vi "Animal Data Processor.vi"() -> (0 "Data Export":T1 {"Data Channels" format="%.2f"})   [LabVIEW 2016]
uses:
  Animal Data Processor state.ctl
  <vilib>/regexp/Match Regular Expression.xnode
panel:
  in  "Case Constant\n(See Context Help)":bool
  in  "Number of Impulse Files":i32
  in  "Field Strengths":i32[](array[numeric])=[1, 2, 7, 8, 13, 14, 20]
  in  "Impulse Data File (auto increment)":bool
  in  "Field Gains from File":bool
  in  "All Data":T1 {"Data Channels" format="%.2f"}
  in  "Tab Control":enum32{"Channel Information", "Default Values"}(tab)
  in  "Defaults":bool
  in  "Coil Combinations":T2(array[cluster])=[{"Direction Coil"=0, "Torsion Coil"=0, "Dir"=FALSE, "tor"=FALSE}, {"Direction Coil"=0, "Torsion Coil"=2, "Dir"=TRUE, "tor"=TRUE}, {"Direction Coil"=2, "Torsion Coil"=3, "Dir"=TRUE, "tor"=TRUE}]
  in  "Coil Information":T3(array[cluster])=[{"X Field"={"Channel No."=2, "Peak Field "=911, "Offset"=0.0, "Gain"=0.0625}, "Y Field"={"Channel No."=0, "Peak Field "=-904, "Offset"=0.0, "Gain"=0.0625}, "Z Field"={"Channel No."=1, "Peak Field "=961, "Offset"=0.0, "Gain"=0.0625}}, {"X Field"={"Channel No."=5, "Peak Field "=770, "Offset"=0.0, "Gain"=0.0625}, "Y Field"={"Channel No."=3, "Peak Field "=-723, "Offset"=0.0, "Gain"=0.0625}, "Z Field"={"Channel No."=4, "Peak Field "=771, "Offset"=0.0, "Gain"=0.0625}}, {"X Field"={"Channel No."=8, "Peak Field "=603, "Offset"=0.0, "Gain"=0.0625}, "Y Field"={"Channel No."=6, "Peak Field "=-647, "Offset"=0.0, "Gain"=0.0625}, "Z Field"={"Channel No."=7, "Peak Field "=627, "Offset"=0.0, "Gain"=0.0625}}, {"X Field"={"Channel No."=11, "Peak Field "=1030, "Offset"=0.0, "Gain"=0.0625}, "Y Field"={"Channel No."=9, "Peak Field "=-1108, "Offset"=0.0, "Gain"=0.0625}, "Z Field"={"Channel No."=10, "Peak Field "=1074, "Offset"=0.0, "Gain"=0.0625}}] {"Z Field"."Gain" format="%.4f"; "Z Field"."Offset" format="%.2f"; "Y Field"."Gain" format="%.4f"; "Y Field"."Offset" format="%.2f"; "X Field"."Gain" format="%.4f"; "X Field"."Offset" format="%.2f"}
  in  "Additional Channels":T4(array[cluster])=[{"Channel No."=12, "Scaling Factor"=0.00030518, "Channel Name"=0, "Offset Factor"=0, "Acutrol Cal"=20}, {"Channel No."=13, "Scaling Factor"=0.00030518, "Channel Name"=1, "Offset Factor"=0, "Acutrol Cal"=20}, {"Channel No."=14, "Scaling Factor"=0.00030518, "Channel Name"=2, "Offset Factor"=0, "Acutrol Cal"=20}, {"Channel No."=15, "Scaling Factor"=0.00030518, "Channel Name"=3, "Offset Factor"=0, "Acutrol Cal"=20}] {"Acutrol Cal" min=0 max=40 step=20; "Channel Name" items=["Chair Position", "Chair Velocity", "Sled Position", "Sled Velocity"]; "Scaling Factor" format="%.4e"}
  in  "Available Channel Names":string[](array[string])=["Chair Position", "Chair Velocity", "Sled Position", "Sled Velocity"]
  in  "Data File":T5 {"Data -> Additional" format="%.2f"; "Data -> 3D Coil" format="%.2f"}
  in  "For DY DZ  (H LE RE) plot\n                 Channel No.":i32[](array[numeric])=[1, 2, 7, 8, 13, 14, 18]
  in  "Export Channel List":u16[](array[ring])=[3, 4, 5, 14, 15, 16, 17, 18, 29, 30, 31, 32, 33, 6, 7, 8, 19, 20, 21, 22, 23, 34, 35, 36, 37, 38, 39, 40, 41, 42, 43] items=["Hx Position-in-Space", "Hy Position-in-Space", "Hz Position-in-Space", "Lx Position-in-Space", "Ly Position-in-Space", "Lz Position-in-Space", "Rx Position-in-Space", "Ry Position-in-Space", "Rz Position-in-Space", "Hx Velocity-in-Space", "Hy Velocity-in-Space", "Hz Velocity-in-Space", "Hl Velocity-in-Space", "Hr Velocity-in-Space", "Lx Velocity-in-Space", "Ly Velocity-in-Space", "Lz Velocity-in-Space", "Ll Velocity-in-Space", "Lr Velocity-in-Space", "Rx Velocity-in-Space", "Ry Velocity-in-Space", "Rz Velocity-in-Space", "Rl Velocity-in-Space", "Rr Velocity-in-Space", "Hx Acceleration-in-Space", "Hy Acceleration-in-Space", "Hz Acceleration-in-Space", "Hl Acceleration-in-Space", "Hr Acceleration-in-Space", "Lx Acceleration-in-Space", "Ly Acceleration-in-Space", "Lz Acceleration-in-Space", "Ll Acceleration-in-Space", "Lr Acceleration-in-Space", "Rx Acceleration-in-Space", "Ry Acceleration-in-Space", "Rz Acceleration-in-Space", "Rl Acceleration-in-Space", "Rr Acceleration-in-Space", "Chair Position", "Chair Velocity", "Sled Position", "Sled Velocity", " "]
  out "Processing":bool
  in  "Start Processing":bool
  in  "Selected Data File":string
  in  "Data File":bool
  in  "Quit":bool
  in  "Stop":bool
  # "Animal Data Processor"
  # "AAM 10 april 2002 ver.10"
  # "Copyright Americo A. Migliaccio (c) 2002 All Rights Reserved by Author"
  # "NOTE: EMPTY LIST ALWAYS AT END"
  # "Head 0; Left Eye 1; Right Eye 2"
  # "Name                        Channel            Offset            Gain               Acutrol Cal"
  # "Channel            Field               Offset             Gain"
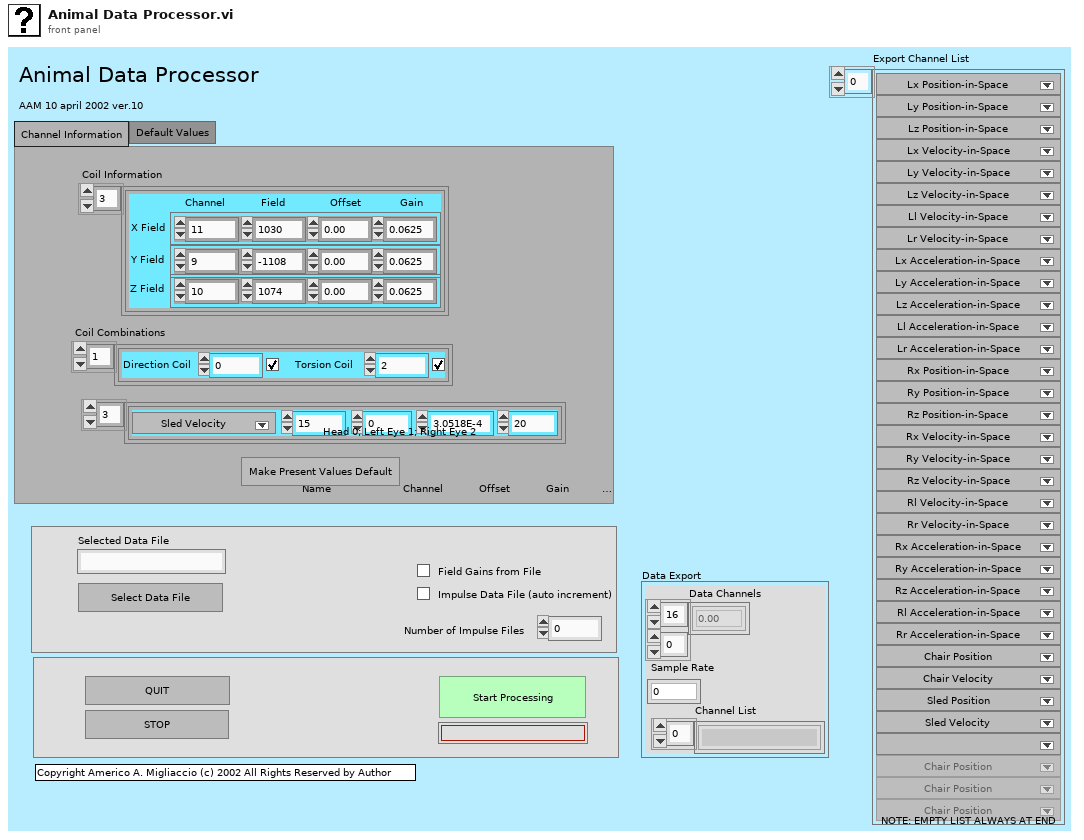
[diagram p1: front panel]
types:
  T1 = cluster{"Data Channels":dbl[][], "Sample Rate":i32, "Channel List":string[]}
  T2 = cluster{"Direction Coil":i32, "Torsion Coil":i32, "Dir":bool, "tor":bool}[]
  T3 = cluster{"X Field":cluster{"Channel No.":i32, "Peak Field ":i32, "Offset":dbl, "Gain":dbl}, "Y Field":cluster{"Channel No.":i32, "Peak Field ":i32, "Offset":dbl, "Gain":dbl}, "Z Field":cluster{"Channel No.":i32, "Peak Field ":i32, "Offset":dbl, "Gain":dbl}}[]
  T4 = cluster{"Channel No.":i32, "Scaling Factor":dbl, "Channel Name":u16, "Offset Factor":i32, "Acutrol Cal":i32}[]
  T5 = cluster{"No. Channels":i32, "Sample Rate":i32, "Data -> 3D Coil":dbl[][], "Data -> Additional":dbl[][]}
  T6 = typedef "Animal Data Processor state.ctl" = enum16{"Calculate 6 Field/Int Rot Matrix", "Panel Monitoring", "Initialize", "Read 6 Field/Int Calibration File", "Read 6 Field/Int Data File", "Sort 6 Field/Int Channels", "Export Channels", "Stop", "Quit"}
  T7 = enum16{"open", "open or create", "create or replace", "create", "open (read only)"}
  T8 = enum16{"Position in Space", "Position in Head", "Position in Eye", "Velocity in Space", "Velocity in Head", "Velocity in Eye", "Acceleration in Space", "Acceleration in Head"}
  T9 = cluster{"Coil Information":cluster{"X Field":cluster{"Channel No.":i32, "Peak Field ":i32, "Offset":dbl, "Gain":dbl}, "Y Field":cluster{"Channel No.":i32, "Peak Field ":i32, "Offset":dbl, "Gain":dbl}, "Z Field":cluster{"Channel No.":i32, "Peak Field ":i32, "Offset":dbl, "Gain":dbl}}[], "Coil Combinations":cluster{"Direction Coil":i32, "Torsion Coil":i32, "Dir":bool, "tor":bool}[], "Additional Channels":cluster{"Channel No.":i32, "Scaling Factor":dbl, "Channel Name":u16, "Offset Factor":i32, "Acutrol Cal":i32}[], "Selected Data File":string, "Data File":cluster{"No. Channels":i32, "Sample Rate":i32, "Data -> 3D Coil":dbl[][], "Data -> Additional":dbl[][]}, "For DY DZ  (H LE RE) plot\n                 Channel No.":i32[], "All Data":cluster{"Data Channels":dbl[][], "Sample Rate":i32, "Channel List":string[]}, "Field Strengths":i32[]}
  T10 = cluster{"Stop ":bool, "Quit":bool, "Data File":bool, "Start Processing":bool, "Defaults":bool}
  T11 = cluster{"Coil Information":cluster{"X Field":cluster{"Channel No.":i32, "Peak Field ":i32, "Offset":dbl, "Gain":dbl}, "Y Field":cluster{"Channel No.":i32, "Peak Field ":i32, "Offset":dbl, "Gain":dbl}, "Z Field":cluster{"Channel No.":i32, "Peak Field ":i32, "Offset":dbl, "Gain":dbl}}[], "Coil Combinations":cluster{"Direction Coil":i32, "Torsion Coil":i32, "Dir":bool, "tor":bool}[], "Additional Channels":cluster{"Channel No.":i32, "Scaling Factor":dbl, "Channel Name":u16, "Offset Factor":i32, "Acutrol Cal":i32}[]}
  T12 = cluster{"X Field":cluster{"Channel No.":i32, "Peak Field ":i32, "Offset":dbl, "Gain":dbl}, "Y Field":cluster{"Channel No.":i32, "Peak Field ":i32, "Offset":dbl, "Gain":dbl}, "Z Field":cluster{"Channel No.":i32, "Peak Field ":i32, "Offset":dbl, "Gain":dbl}}
  T13 = enum16{"Rotation Matrix", "Rotation Vectors", "Quaternions", "Fick Angles", "Helmholtz Angles"}
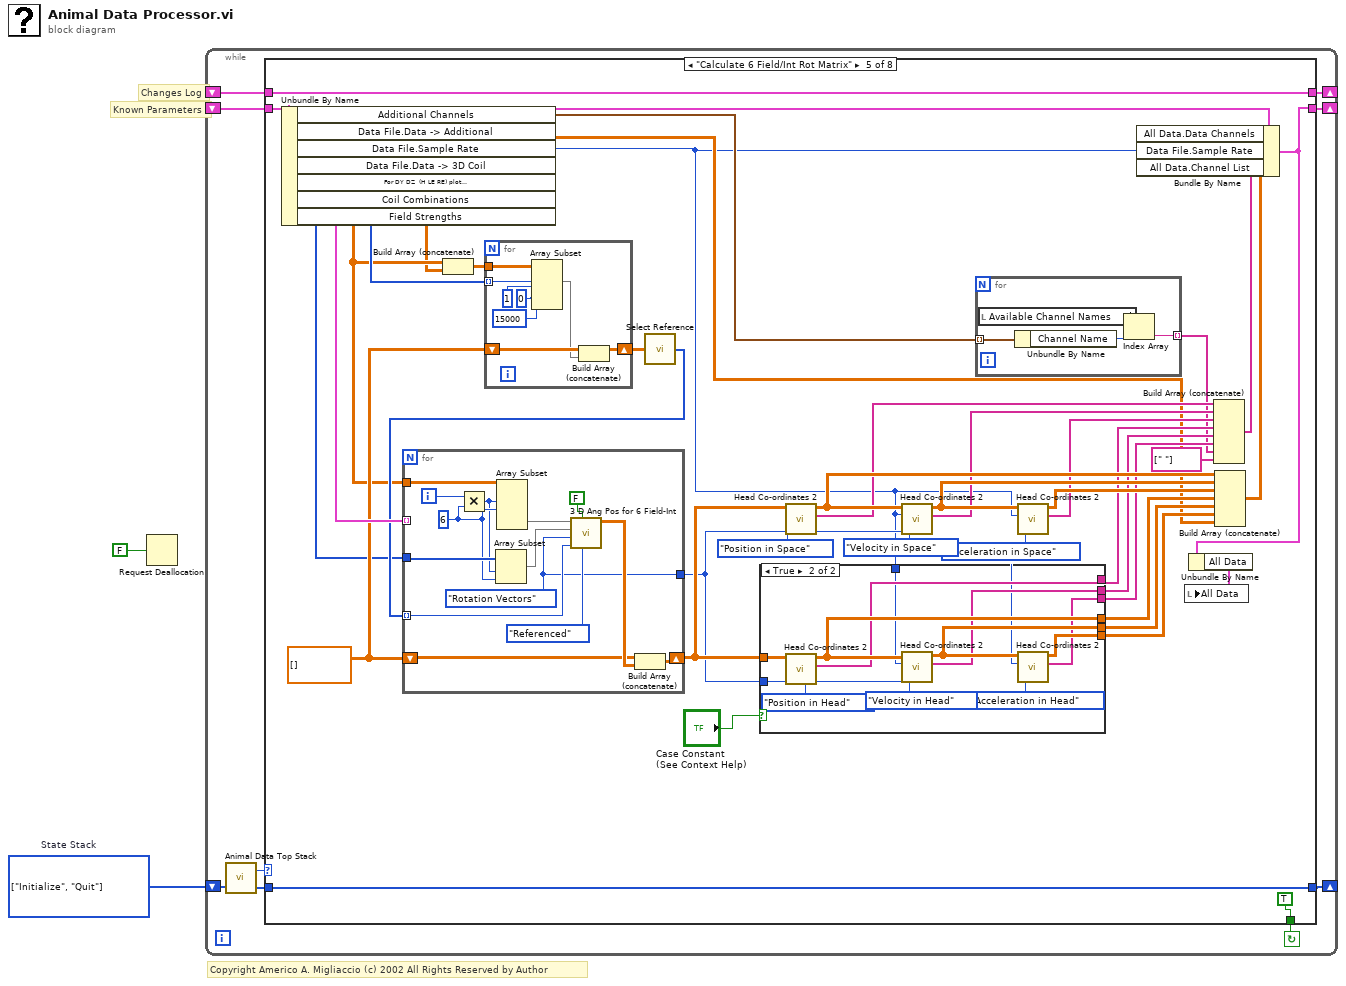
[diagram p0: block diagram]
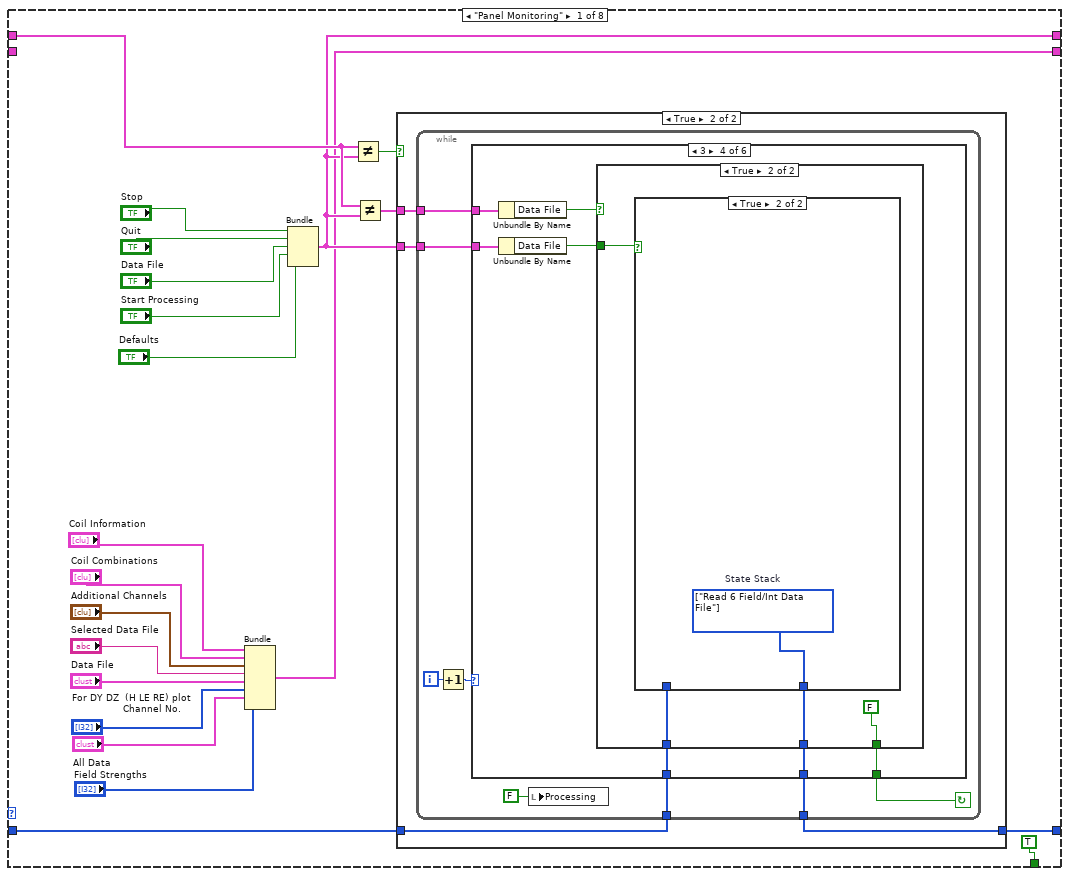
[diagram p2: hidden frame]
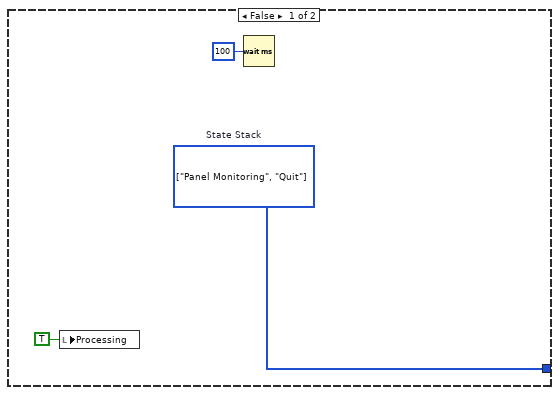
[diagram p3: hidden frame]
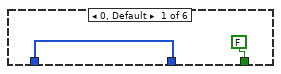
[diagram p4: hidden frame]
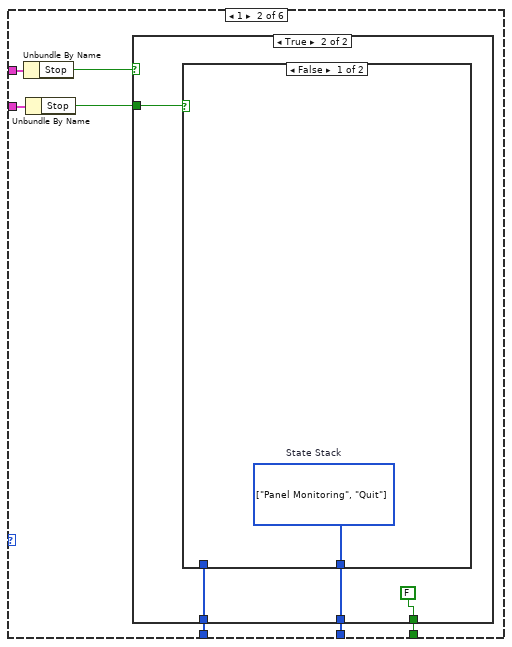
[diagram p5: hidden frame]
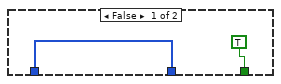
[diagram p6: hidden frame]
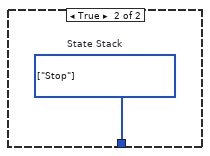
[diagram p7: hidden frame]
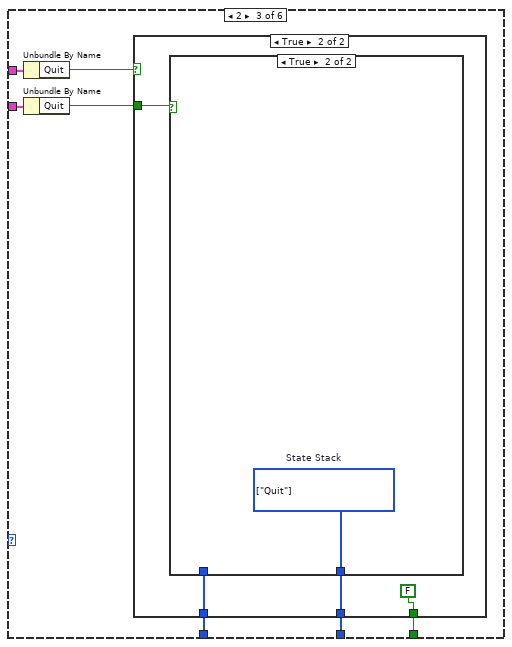
[diagram p8: hidden frame]
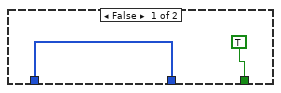
[diagram p9: hidden frame]
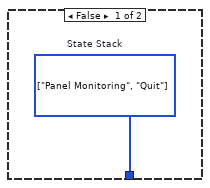
[diagram p10: hidden frame]
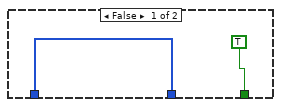
[diagram p11: hidden frame]
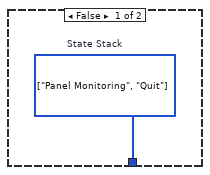
[diagram p12: hidden frame]
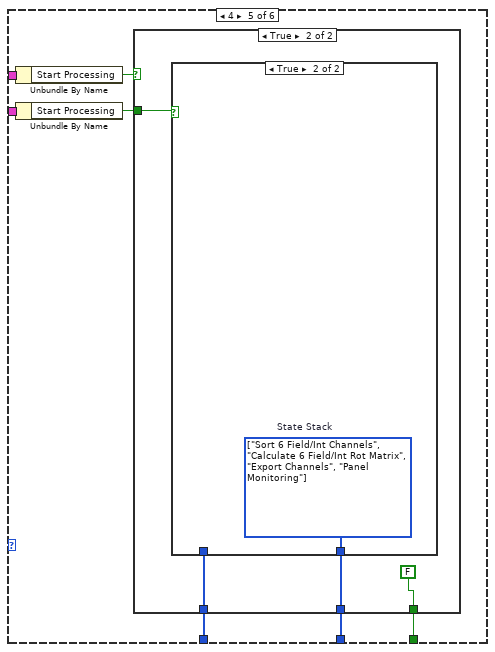
[diagram p13: hidden frame]
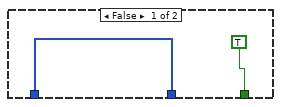
[diagram p14: hidden frame]
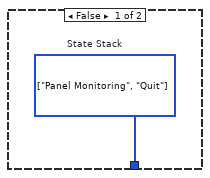
[diagram p15: hidden frame]
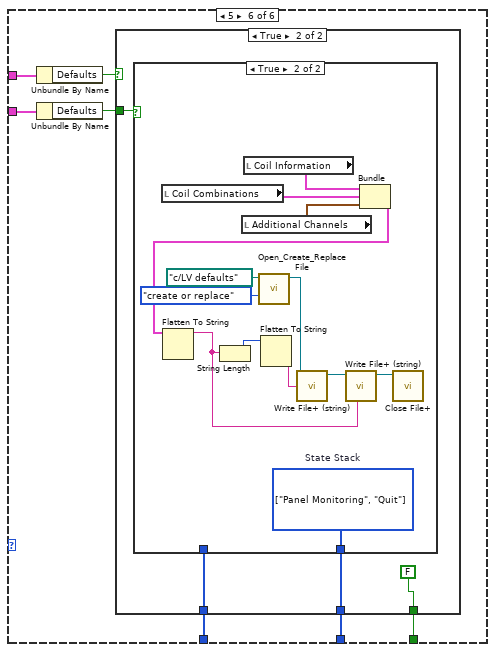
[diagram p16: hidden frame]
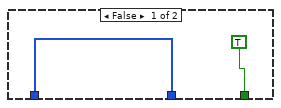
[diagram p17: hidden frame]
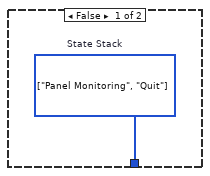
[diagram p18: hidden frame]
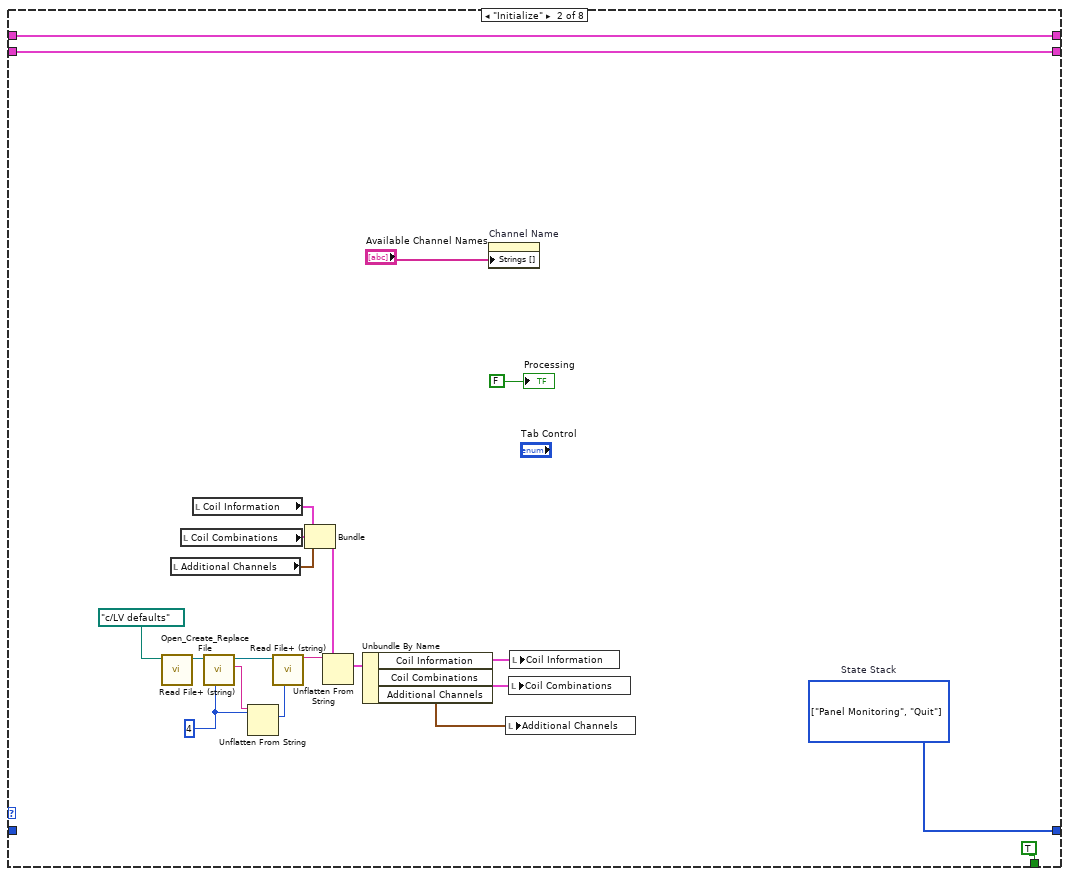
[diagram p19: hidden frame]
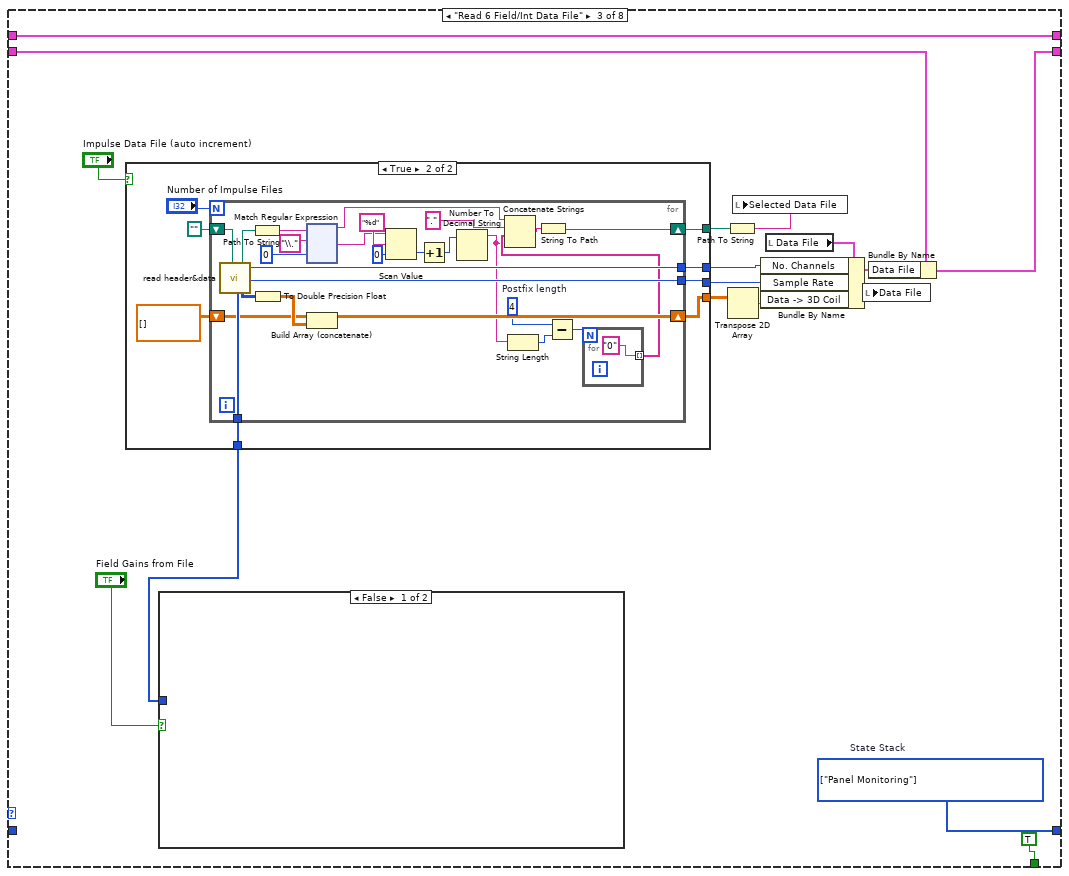
[diagram p20: hidden frame]
diagram:
  w2 = T6[] [enum."Initialize", enum."Quit"] items=["Calculate 6 Field/Int Rot Matrix", "Panel Monitoring", "Initialize", "Read 6 Field/Int Calibration File", "Read 6 Field/Int Data File", "Sort 6 Field/Int Channels", "Export Channels", "Stop", "Quit"]  # State Stack
  # "Copyright Americo A. Migliaccio (c) 2002 All Rights Reserved by Author"
  # "Known Parameters"
  # "Changes Log"
  n1 = Request Deallocation(FALSE ("flag")) -> ()
  n2 = while {
    shift-left: _ -> [w4]
    shift-right: [w3] -> _
    shift-left: _ -> [w6]
    shift-right: [w7] -> _
    shift-left: w2 -> [w11]
    shift-right: [w9] -> _
    stop <- w5 continue-if-true
    n3 = call "Animal Data Top Stack.vi"("State Stack (in)"=w11) -> ("State Stack (out)"=w10:T6[], "State"=w8:T6)  [unwired: 1 in]
    n4 = case shown="\"Calculate 6 Field/Int Rot Matrix\"" w8 {
      tunnel: w10 -> [w27 _ _ w353 w489 w541 w550 w554]
      tunnel: [w26 w153 w169 w353 w489 w541 w550 w554] -> w9
      tunnel: [w24 w156 w172 w355 w487 w539 w548 w552] -> w7
      tunnel: w6 -> [w29 w156 w172 w355 w487 w539 w548 w552]
      tunnel: [TRUE TRUE TRUE TRUE TRUE FALSE FALSE FALSE] -> w5
      tunnel: [w12 w145 w171 w352 w471 w535 w547 w551] -> w3
      tunnel: w4 -> [_ w145 w170 w354 w481 w535 w547 w551]
      frame "Panel Monitoring" {
        n5 = Bundle("Coil Information"="Coil Information", "Coil Combinations"="Coil Combinations", "Additional Channels"="Additional Channels", "Selected Data File"="Selected Data File", "Data File"="Data File", "For DY DZ  (H LE RE) plot\n                 Channel No."="For DY DZ  (H LE RE) plot\n                 Channel No.", "All Data"="All Data", "Field Strengths"="Field Strengths") -> (w12:T9)  [unwired: 1 in]
        n6 = Bundle("Stop"="Stop", "Quit"="Quit", "Data File"="Data File", "Start Processing"="Start Processing", "Defaults"="Defaults") -> (w24:T10)  [unwired: 1 in]
        n7 = Not Equal?(x=w29, y=w24) -> (x != y?=w30:bool)
        n8 = Not Equal?(x=w29, y=w24) -> (x != y?=w28:T10)
        n9 = case shown="True" w30 {
          tunnel: w28 -> [_ w39]
          tunnel: w27 -> [_ w37]
          tunnel: [w33 w38] -> w26
          tunnel: w24 -> [_ w36]
          frame False {
            w33 = T6[] [enum."Panel Monitoring", enum."Quit"] items=["Calculate 6 Field/Int Rot Matrix", "Panel Monitoring", "Initialize", "Read 6 Field/Int Calibration File", "Read 6 Field/Int Data File", "Sort 6 Field/Int Channels", "Export Channels", "Stop", "Quit"]  # State Stack
            n10 = local write "Processing"(TRUE ("Processing")) -> ()
            n11 = Wait (ms)(milliseconds to wait=u32 100) -> ()  [unwired: 1 out]
          }
          frame True {
            n12 = while {
              tunnel: w36 -> [w41]
              tunnel: w37 -> [w44]
              tunnel: [w45] -> w38
              tunnel: w39 -> [w47]
              i -> [w46]
              stop <- w43 continue-if-true
              n13 = Increment(x=w46) -> (x+1=w42:i32)
              n14 = case shown="3" w42 {
                tunnel: w47 -> [_ w56 w71 w86 w101 w116]
                tunnel: [w49 w54 w69 w84 w99 w114] -> w45
                tunnel: w44 -> [w49 w53 w68 w83 w98 w113]
                tunnel: [FALSE w52 w67 w82 w97 w112] -> w43
                tunnel: w41 -> [_ w51 w66 w81 w96 w111]
                frame 0, Default {
                }
                frame 1 {
                  n15 = Unbundle By Name(w56) -> ("Stop"=w55:bool)
                  n16 = Unbundle By Name(w51) -> ("Stop"=w50:bool)
                  n17 = case shown="True" w55 {
                    tunnel: [w58 w62] -> w54
                    tunnel: w53 -> [w58 w60]
                    tunnel: [TRUE FALSE] -> w52
                    tunnel: w50 -> [_ w61]
                    frame False {
                    }
                    frame True {
                      n18 = case shown="False" w61 {
                        tunnel: [w63 w64] -> w62
                        tunnel: w60 -> [_ _]
                        frame False {
                          w63 = T6[] [enum."Panel Monitoring", enum."Quit"] items=["Calculate 6 Field/Int Rot Matrix", "Panel Monitoring", "Initialize", "Read 6 Field/Int Calibration File", "Read 6 Field/Int Data File", "Sort 6 Field/Int Channels", "Export Channels", "Stop", "Quit"]  # State Stack
                        }
                        frame True {
                          w64 = T6[] [enum."Stop"] items=["Calculate 6 Field/Int Rot Matrix", "Panel Monitoring", "Initialize", "Read 6 Field/Int Calibration File", "Read 6 Field/Int Data File", "Sort 6 Field/Int Channels", "Export Channels", "Stop", "Quit"]  # State Stack
                        }
                      }
                    }
                  }
                }
                frame 2 {
                  n19 = Unbundle By Name(w71) -> ("Quit"=w70:bool)
                  n20 = Unbundle By Name(w66) -> ("Quit"=w65:bool)
                  n21 = case shown="True" w70 {
                    tunnel: [w73 w77] -> w69
                    tunnel: w68 -> [w73 w75]
                    tunnel: [TRUE FALSE] -> w67
                    tunnel: w65 -> [_ w76]
                    frame False {
                    }
                    frame True {
                      n22 = case shown="True" w76 {
                        tunnel: [w78 w79] -> w77
                        tunnel: w75 -> [_ _]
                        frame False {
                          w78 = T6[] [enum."Panel Monitoring", enum."Quit"] items=["Calculate 6 Field/Int Rot Matrix", "Panel Monitoring", "Initialize", "Read 6 Field/Int Calibration File", "Read 6 Field/Int Data File", "Sort 6 Field/Int Channels", "Export Channels", "Stop", "Quit"]  # State Stack
                        }
                        frame True {
                          w79 = T6[] [enum."Quit"] items=["Calculate 6 Field/Int Rot Matrix", "Panel Monitoring", "Initialize", "Read 6 Field/Int Calibration File", "Read 6 Field/Int Data File", "Sort 6 Field/Int Channels", "Export Channels", "Stop", "Quit"]  # State Stack
                        }
                      }
                    }
                  }
                }
                frame 3 {
                  n23 = Unbundle By Name(w86) -> ("Data File"=w85:bool)
                  n24 = Unbundle By Name(w81) -> ("Data File"=w80:bool)
                  n25 = case shown="True" w85 {
                    tunnel: [w88 w92] -> w84
                    tunnel: w83 -> [w88 w91]
                    tunnel: [TRUE FALSE] -> w82
                    tunnel: w80 -> [_ w90]
                    frame False {
                    }
                    frame True {
                      n26 = case shown="True" w90 {
                        tunnel: [w93 w94] -> w92
                        tunnel: w91 -> [_ _]
                        frame False {
                          w93 = T6[] [enum."Panel Monitoring", enum."Quit"] items=["Calculate 6 Field/Int Rot Matrix", "Panel Monitoring", "Initialize", "Read 6 Field/Int Calibration File", "Read 6 Field/Int Data File", "Sort 6 Field/Int Channels", "Export Channels", "Stop", "Quit"]  # State Stack
                        }
                        frame True {
                          w94 = T6[] [enum."Read 6 Field/Int Data File"] items=["Calculate 6 Field/Int Rot Matrix", "Panel Monitoring", "Initialize", "Read 6 Field/Int Calibration File", "Read 6 Field/Int Data File", "Sort 6 Field/Int Channels", "Export Channels", "Stop", "Quit"]  # State Stack
                        }
                      }
                    }
                  }
                }
                frame 4 {
                  n27 = Unbundle By Name(w101) -> ("Start Processing"=w100:bool)
                  n28 = Unbundle By Name(w96) -> ("Start Processing"=w95:bool)
                  n29 = case shown="True" w100 {
                    tunnel: [w103 w107] -> w99
                    tunnel: w98 -> [w103 w106]
                    tunnel: [TRUE FALSE] -> w97
                    tunnel: w95 -> [_ w105]
                    frame False {
                    }
                    frame True {
                      n30 = case shown="True" w105 {
                        tunnel: [w108 w109] -> w107
                        tunnel: w106 -> [_ _]
                        frame False {
                          w108 = T6[] [enum."Panel Monitoring", enum."Quit"] items=["Calculate 6 Field/Int Rot Matrix", "Panel Monitoring", "Initialize", "Read 6 Field/Int Calibration File", "Read 6 Field/Int Data File", "Sort 6 Field/Int Channels", "Export Channels", "Stop", "Quit"]  # State Stack
                        }
                        frame True {
                          w109 = T6[] [enum."Sort 6 Field/Int Channels", enum."Calculate 6 Field/Int Rot Matrix", enum."Export Channels", enum."Panel Monitoring"] items=["Calculate 6 Field/Int Rot Matrix", "Panel Monitoring", "Initialize", "Read 6 Field/Int Calibration File", "Read 6 Field/Int Data File", "Sort 6 Field/Int Channels", "Export Channels", "Stop", "Quit"]  # State Stack
                        }
                      }
                    }
                  }
                }
                frame 5 {
                  n31 = Unbundle By Name(w116) -> ("Defaults"=w115:bool)
                  n32 = Unbundle By Name(w111) -> ("Defaults"=w110:bool)
                  n33 = case shown="True" w115 {
                    tunnel: [w118 w122] -> w114
                    tunnel: w113 -> [w118 w121]
                    tunnel: [TRUE FALSE] -> w112
                    tunnel: w110 -> [_ w120]
                    frame False {
                    }
                    frame True {
                      n34 = case shown="True" w120 {
                        tunnel: [w123 w136] -> w122
                        tunnel: w121 -> [_ _]
                        frame False {
                          w123 = T6[] [enum."Panel Monitoring", enum."Quit"] items=["Calculate 6 Field/Int Rot Matrix", "Panel Monitoring", "Initialize", "Read 6 Field/Int Calibration File", "Read 6 Field/Int Data File", "Sort 6 Field/Int Channels", "Export Channels", "Stop", "Quit"]  # State Stack
                        }
                        frame True {
                          w136 = T6[] [enum."Panel Monitoring", enum."Quit"] items=["Calculate 6 Field/Int Rot Matrix", "Panel Monitoring", "Initialize", "Read 6 Field/Int Calibration File", "Read 6 Field/Int Data File", "Sort 6 Field/Int Channels", "Export Channels", "Stop", "Quit"]  # State Stack
                          n35 = local read "Coil Combinations"() -> (w126:T2)
                          n36 = local read "Additional Channels"() -> (w125:T4)
                          n37 = local read "Coil Information"() -> (w127:T3)
                          n38 = call <vilib>:"Open_Create_Replace File.vi"("function (open:0)"=T7."create or replace", "file path"=path "c:/LV defaults") -> ("refnum"=w129:refnum<file>)  [unwired: 6 in, 3 out]
                          n39 = Bundle("Coil Information"=w127, "Coil Combinations"=w126, "Additional Channels"=w125) -> (w124:T11)  [unwired: 1 in]
                          n40 = Flatten To String(anything=w124) -> (data string=w131:string)  [unwired: 3 in, 2 out]
                          n41 = String Length(string=w131) -> (length=w133:i32)
                          n42 = Flatten To String(anything=w133) -> (data string=w132:string)  [unwired: 3 in, 2 out]
                          n43 = call <vilib>:"Write File+ (string).vi"("string"=w132, "refnum"=w129) -> ("dup refnum"=w130:refnum<file>)  [unwired: 5 in, 2 out]
                          n44 = call <vilib>:"Write File+ (string).vi"("string"=w131, "refnum"=w130) -> ("dup refnum"=w135:refnum<file>)  [unwired: 5 in, 2 out]
                          n45 = call <vilib>:"Close File+.vi"("refnum"=w135) -> ()  [unwired: 4 in, 3 out]
                        }
                      }
                    }
                  }
                }
              }
              n46 = local write "Processing"(FALSE ("Processing")) -> ()
            }
          }
        }
      }
      frame "Initialize" {
        w153 = T6[] [enum."Panel Monitoring", enum."Quit"] items=["Calculate 6 Field/Int Rot Matrix", "Panel Monitoring", "Initialize", "Read 6 Field/Int Calibration File", "Read 6 Field/Int Data File", "Sort 6 Field/Int Channels", "Export Channels", "Stop", "Quit"]  # State Stack
        w148 = 4 ("count")
        n47 = call <vilib>:"Open_Create_Replace File.vi"("file path"=path "c:/LV defaults") -> ("refnum"=w151:refnum<file>)  [unwired: 7 in, 3 out]
        n48 = local read "Additional Channels"() -> (w142:T4)
        n49 = local read "Coil Combinations"() -> (w143:T2)
        n50 = local read "Coil Information"() -> (w144:T3)
        n51 = call <vilib>:"Read File+ (string).vi"("count"=w148, "refnum"=w151) -> ("string"=w149:string, "dup refnum"=w150:refnum<file>)  [unwired: 5 in, 3 out]
        n52 = Unflatten From String(type=w148, binary string=w149) -> (value=w147:i32)  [unwired: 3 in, 2 out]
        n53 = call <vilib>:"Read File+ (string).vi"("count"=w147, "refnum"=w150) -> ("string"=w152:string)  [unwired: 5 in, 4 out]
        n54 = Bundle("Coil Information"=w144, "Coil Combinations"=w143, "Additional Channels"=w142) -> (w141:T11)  [unwired: 1 in]
        n55 = Unflatten From String(type=w141, binary string=w152) -> (value=w140:T11)  [unwired: 3 in, 2 out]
        n56 = Unbundle By Name(w140) -> ("Coil Information"=w138:T3, "Coil Combinations"=w139:T2, "Additional Channels"=w137:T4)
        n57 = property on="Channel Name" class="Ring (strict)"("Strings []"="Available Channel Names") -> ()  [unwired: 2 in, 2 out]
        n58 = local write "Additional Channels"(w137) -> ()
        n59 = local write "Coil Combinations"(w139) -> ()
        n60 = local write "Coil Information"(w138) -> ()
        "Processing" <- FALSE ("Processing")
      }
      frame "Read 6 Field/Int Data File" {
        w169 = T6[] [enum."Panel Monitoring"] items=["Calculate 6 Field/Int Rot Matrix", "Panel Monitoring", "Initialize", "Read 6 Field/Int Calibration File", "Read 6 Field/Int Data File", "Sort 6 Field/Int Channels", "Export Channels", "Stop", "Quit"]  # State Stack
        n61 = case shown="True" "Impulse Data File (auto increment)" {
          tunnel: [w175 w185] -> w164
          tunnel: [w176 w186] -> w163
          tunnel: [w178 w182] -> w159
          tunnel: [w177 w187] -> w162
          tunnel: [w174 w181] -> w161
          frame False {
            n62 = call "read header&data.vi"() -> ("numchans"=w175:i32, "ADD1"=w176:i32, "Field strength"=w177:i32[], "Data Array"=w179:i16[][], "path(out)"=w174:path)  [unwired: 4 in, 11 out]
            n63 = To Double Precision Float(number=w179) -> (double precision float=w178:dbl[][])
          }
          frame True {
            n64 = for {
              N: "Number of Impulse Files" -> [_]
              tunnel: [w212] -> w187
              tunnel: [w211] -> w186
              tunnel: [w210] -> w185
              shift-right: [w208] -> w182
              shift-left: dbl[][] [] -> [w207]
              shift-right: [w199] -> w181
              shift-left: path "" -> [w206]
              w194 = 4  # Postfix length
              n65 = call "read header&data.vi"("file path(in)"=w206) -> ("numchans"=w210:i32, "ADD1"=w211:i32, "Field strength"=w212:i32[], "Data Array"=w213:i16[][], "path(out)"=w205:path)  [unwired: 3 in, 11 out]
              n66 = Path To String(path=w205) -> (string=w188:string)
              n67 = To Double Precision Float(number=w213) -> (double precision float=w209:dbl[][])
              n68 = xnode "Match Regular Expression"("input string"=w188, "regular expression"="\\.", "offset (0)"=0) -> ("before match"=w196:string, "after match"=w197:string)  [unwired: 3 in, 3 out]
              n69 = Build Array (concatenate)(w207, w209) -> (w208:dbl[][])
              n70 = Scan Value(string=w197, format string="%d", default (0 dbl)=0) -> (value=w203:i32)  [unwired: 1 out]
              n71 = Increment(x=w203) -> (x+1=w201:i32)
              n72 = Number To Decimal String(number=w201) -> (decimal integer string=w191:string)  [unwired: 1 in]
              n73 = String Length(string=w191) -> (length=w195:i32)
              n74 = Subtract(x=w194, y=w195) -> (x-y=w193:i32)
              n75 = for {
                N: w193 -> [_]
                tunnel: ["0"] -> w192 mode=indexing
              }
              n76 = Concatenate Strings(w196, "." ("string"), w192, w191) -> (w200:string)
              n77 = String To Path(string=w200) -> (path=w199:path)
            }
          }
        }
        n78 = case shown="False" "Field Gains from File" {
          tunnel: w162 -> [_ w329]
          frame False {
          }
          frame True {
            n79 = local read "Coil Information"() -> (w326:T3)
            n80 = Array Size(array=w326) -> (size(s)=w328:i32)
            n81 = for {
              tunnel: w326 -> [w340] mode=indexing
              tunnel: w329 -> [w334]
              tunnel: w328 -> [w338]
              tunnel: [w333] -> w327 mode=indexing
              i -> [w339]
              n82 = Multiply(x=w338, y=w339) -> (x*y=w337:i32)
              n83 = Increment(x=w337) -> (x+1=w335:i32)
              n84 = Increment(x=w335) -> (x+1=w336:i32)
              n85 = Index Array(array=w334, index=w337) -> (element=w330:i32)
              n86 = Index Array(array=w334, index=w335) -> (element=w331:i32)
              n87 = Index Array(array=w334, index=w336) -> (element=w332:i32)
              n88 = Bundle By Name(cluster=w340, "X Field.Peak Field"=w330, "Y Field.Peak Field"=w331, "Z Field.Peak Field"=w332) -> (w333:T12)
            }
            n89 = local write "Coil Information"(w327) -> ()
          }
        }
        n90 = Path To String(path=w161) -> (string=w160:string)
        n91 = Transpose 2D Array(2D array=w159) -> (transposed array=w158:dbl[][])
        n92 = local write "Selected Data File"(w160) -> ()
        n93 = local read "Data File"() -> (w168:T5)
        n94 = Bundle By Name(cluster=w168, "No. Channels"=w164, "Sample Rate"=w163, "Data -> 3D Coil"=w158) -> (w166:T5)
        n95 = local write "Data File"(w166) -> ()
        n96 = Bundle By Name(cluster=w170, "Data File"=w166) -> (w171:T9)
      }
      frame "Sort 6 Field/Int Channels" {
        w344 = dbl[][] []
        n97 = Unbundle By Name(w354) -> ("Data File.Data -> 3D Coil"=w345:dbl[][])
        n98 = local read "Additional Channels"() -> (w346:T4)
        n99 = local read "Coil Combinations"() -> (w349:T2)
        n100 = local read "Coil Information"() -> (w348:T3)
        n101 = for {
          tunnel: w349 -> [w400] mode=indexing
          tunnel: w348 -> [w398]
          tunnel: w345 -> [w380]
          shift-right: [w391] -> w347
          shift-left: w344 -> [w390]
          shift-right: [w383] -> w341
          shift-left: i32[] [] -> [w384]
          n102 = Unbundle By Name(w400) -> ("Dir"=w381:bool, "Direction Coil"=w399:i32, "Torsion Coil"=w397:i32, "tor"=w395:bool)
          n103 = Index Array(array=w398, index=w399) -> (element=w382:T12)
          n104 = Index Array(array=w398, index=w397) -> (element=w396:T12)
          n105 = case shown="True" w381 {
            tunnel: w382 -> [_ w406]
            tunnel: w380 -> [_ w410]
            tunnel: [w402 w409] -> w377
            tunnel: [w402 w408] -> w378
            tunnel: [w402 w407] -> w379
            tunnel: [w401 w405] -> w374
            tunnel: [w401 w404] -> w376
            tunnel: [w401 w403] -> w375
            frame False {
              w402 = dbl[] [0.0]
              w401 = 1 ("Peak Field")
            }
            frame True {
              n106 = Unbundle By Name(w406) -> ("X Field.Channel No."=w419:i32, "X Field.Offset"=w418:dbl, "X Field.Gain"=w417:dbl, "Y Field.Channel No."=w416:i32, "Y Field.Offset"=w414:dbl, "Y Field.Gain"=w415:dbl, "Z Field.Channel No."=w413:i32, "Z Field.Offset"=w412:dbl, "Z Field.Gain"=w411:dbl)
              n107 = Unbundle By Name(w406) -> ("X Field.Peak Field"=w405:i32, "Y Field.Peak Field"=w404:i32, "Z Field.Peak Field"=w403:i32)
              n108 = Index Array(array=w410, index (row)=w419) -> (element=w423:dbl[])  [unwired: 1 in]
              n109 = Index Array(array=w410, index (row)=w416) -> (element=w424:dbl[])  [unwired: 1 in]
              n110 = Index Array(array=w410, index (row)=w413) -> (element=w425:dbl[])  [unwired: 1 in]
              n111 = Subtract(x=w424, y=w414) -> (x-y=w421:dbl[])
              n112 = Subtract(x=w425, y=w412) -> (x-y=w422:dbl[])
              n113 = Subtract(x=w423, y=w418) -> (x-y=w420:dbl[])
              n114 = Multiply(x=w422, y=w411) -> (x*y=w407:dbl[])
              n115 = Multiply(x=w421, y=w415) -> (x*y=w408:dbl[])
              n116 = Multiply(x=w420, y=w417) -> (x*y=w409:dbl[])
            }
          }
          n117 = case shown="True" w395 {
            tunnel: w396 -> [_ w431]
            tunnel: w380 -> [_ w435]
            tunnel: [w427 w434] -> w394
            tunnel: [w427 w433] -> w393
            tunnel: [w427 w432] -> w392
            tunnel: [w426 w430] -> w388
            tunnel: [w426 w429] -> w387
            tunnel: [w426 w428] -> w386
            frame False {
              w427 = dbl[] [0.0]
              w426 = 1 ("Peak Field")
            }
            frame True {
              n118 = Unbundle By Name(w431) -> ("X Field.Channel No."=w444:i32, "X Field.Offset"=w443:dbl, "X Field.Gain"=w442:dbl, "Y Field.Channel No."=w441:i32, "Y Field.Offset"=w439:dbl, "Y Field.Gain"=w440:dbl, "Z Field.Channel No."=w438:i32, "Z Field.Offset"=w437:dbl, "Z Field.Gain"=w436:dbl)
              n119 = Unbundle By Name(w431) -> ("X Field.Peak Field"=w430:i32, "Y Field.Peak Field"=w429:i32, "Z Field.Peak Field"=w428:i32)
              n120 = Index Array(array=w435, index (row)=w444) -> (element=w448:dbl[])  [unwired: 1 in]
              n121 = Index Array(array=w435, index (row)=w441) -> (element=w449:dbl[])  [unwired: 1 in]
              n122 = Index Array(array=w435, index (row)=w438) -> (element=w450:dbl[])  [unwired: 1 in]
              n123 = Subtract(x=w449, y=w439) -> (x-y=w446:dbl[])
              n124 = Subtract(x=w450, y=w437) -> (x-y=w447:dbl[])
              n125 = Subtract(x=w448, y=w443) -> (x-y=w445:dbl[])
              n126 = Multiply(x=w447, y=w436) -> (x*y=w432:dbl[])
              n127 = Multiply(x=w446, y=w440) -> (x*y=w433:dbl[])
              n128 = Multiply(x=w445, y=w442) -> (x*y=w434:dbl[])
            }
          }
          n129 = Build Array(w377, w378, w379, w394, w393, w392) -> (w389:dbl[][])
          n130 = Build Array (concatenate)(w390, w389) -> (w391:dbl[][])
          n131 = Build Array(w374, w376, w375, w388, w387, w386) -> (w385:i32[])
          n132 = Build Array (concatenate)(w384, w385) -> (w383:i32[])
        }
        n133 = for {
          tunnel: w345 -> [w370]
          shift-right: [w364] -> w343
          shift-left: w344 -> [w365]
          tunnel: w346 -> [w362] mode=indexing
          n134 = Unbundle By Name(w362) -> ("Channel No."=w363:i32, "Offset Factor"=w368:i32, "Scaling Factor"=w367:dbl, "Acutrol Cal"=w358:i32)
          n135 = Equal To 0?(x=w358) -> (x = 0?=w359:bool)
          n136 = Index Array(array=w370, index (row)=w363) -> (element=w369:dbl[])  [unwired: 1 in]
          n137 = case shown="False" w359 {
            tunnel: w358 -> [w371 w373]
            tunnel: [w371 w372] -> w357
            frame False {
            }
            frame True {
              n138 = Increment(x=w373) -> (x+1=w372:i32)
            }
          }
          n139 = Subtract(x=w369, y=w368) -> (x-y=w366:dbl[])
          n140 = Multiply(x=w366, y=w367) -> (x*y=w361:dbl[])
          n141 = Multiply(x=w361, y=w357) -> (x*y=w360:dbl[])
          n142 = Build Array (concatenate)(w365, w360) -> (w364:dbl[][])
        }
        n143 = local read "Data File"() -> (w351:T5)
        n144 = Bundle By Name(cluster=w351, "Data -> 3D Coil"=w347, "Data -> Additional"=w343) -> (w350:T5)
        n145 = local write "Data File"(w350) -> ()
        n146 = local write "Field Strengths"(w341) -> ()
        n147 = Bundle By Name(cluster=w354, "Field Strengths"=w341, "Data File"=w350) -> (w352:T9)
      }
      frame "Calculate 6 Field/Int Rot Matrix" {
        w483 = dbl[][] []
        n148 = Unbundle By Name(w481) -> ("Additional Channels"=w470:T4, "Data File.Data -> Additional"=w458:dbl[][], "Data File.Sample Rate"=w457:i32, "Data File.Data -> 3D Coil"=w469:dbl[][], "For DY DZ  (H LE RE) plot\n                 Channel No."=w486:i32[], "Coil Combinations"=w485:T2, "Field Strengths"=w456:i32[])
        n149 = Build Array (concatenate)(w469, w458) -> (w468:dbl[][])
        n150 = for {
          tunnel: w486 -> [w528] mode=indexing
          tunnel: w468 -> [w529]
          shift-right: [w525] -> w482
          shift-left: w483 -> [w527]
          n151 = Array Subset(array=w529, index (row)=w528, length (row)=1 ("Array Length"), index (col)=0 ("Array Index"), length (col)=15000 ("Array Length")) -> (w526:dbl[][])
          n152 = Build Array (concatenate)(w527, w526) -> (w525:dbl[][])
        }
        n153 = call "Select Reference.vi"("3D Coil"=w482) -> ("References"=w484:i32[])
        n154 = for {
          tunnel: w485 -> [_] mode=indexing
          tunnel: w469 -> [w521]
          tunnel: w456 -> [w512]
          tunnel: w484 -> [w518] mode=indexing
          shift-right: [w516] -> w480
          shift-left: w483 -> [w515]
          tunnel: [w513] -> w479
          i -> [w520]
          w513 = T13."Rotation Vectors" ("3D Convention")
          w511 = 6 ("x")
          n155 = Multiply(x=w520, y=w511) -> (x*y=w510:i32)
          n156 = Array Subset(array=w512, index=w510, length=w511) -> (w509:i32[])
          n157 = Array Subset(array=w521, index (row)=w510, length (row)=w511) -> (w519:dbl[][])  [unwired: 2 in]
          n158 = call "3 D Ang Pos for 6 Field-Int.vi"("With Respect To:"=enum16{"Referenced", "UnReferenced"}."Referenced", "LE and RE 2D coils"=FALSE, "Reference index"=w518, "3D Convention"=w513, "Field Gains"=w509, "3D Voltage Data"=w519) -> ("3D Position"=w517:dbl[][])  [unwired: 5 in]
          n159 = Build Array (concatenate)(w515, w517) -> (w516:dbl[][])
        }
        n160 = case shown="True" "Case Constant\n(See Context Help)" {
          tunnel: w480 -> [_ w503]
          tunnel: w479 -> [_ w502]
          tunnel: [w490 w501] -> w475
          tunnel: [w490 w500] -> w474
          tunnel: [w490 w499] -> w473
          tunnel: [w491 w498] -> w464
          tunnel: [w491 w497] -> w463
          tunnel: [w491 w496] -> w462
          tunnel: w457 -> [_ w495]
          frame False {
            w490 = dbl[][] [] ("3D Output")
            w491 = string[] [] ("Channel List")
          }
          frame True {
            n161 = call "Head Co-ordinates 2.vi"("3D Convention"=w502, "3D Type and Co-ordinate System"=T8."Position in Head", "Array"=w503) -> ("Channel List"=w498:string[], "3D Output"=w501:dbl[][])  [unwired: 3 in]
            n162 = call "Head Co-ordinates 2.vi"("3D Convention"=w502, "3D Type and Co-ordinate System"=T8."Velocity in Head", "Sample Rate"=w495, "Array"=w501) -> ("Channel List"=w497:string[], "3D Output"=w500:dbl[][])  [unwired: 2 in]
            n163 = call "Head Co-ordinates 2.vi"("3D Type and Co-ordinate System"=T8."Acceleration in Head", "Sample Rate"=w495, "Array"=w500) -> ("Channel List"=w496:string[], "3D Output"=w499:dbl[][])  [unwired: 3 in]
          }
        }
        n164 = call "Head Co-ordinates 2.vi"("3D Convention"=w479, "3D Type and Co-ordinate System"=T8."Position in Space", "Array"=w480) -> ("Channel List"=w467:string[], "3D Output"=w478:dbl[][])  [unwired: 3 in]
        n165 = call "Head Co-ordinates 2.vi"("3D Convention"=w479, "3D Type and Co-ordinate System"=T8."Velocity in Space", "Sample Rate"=w457, "Array"=w478) -> ("Channel List"=w466:string[], "3D Output"=w477:dbl[][])  [unwired: 2 in]
        n166 = for {
          tunnel: w470 -> [w507] mode=indexing
          tunnel: [w504] -> w459 mode=indexing
          n167 = local read "Available Channel Names"() -> (w506:string[])
          n168 = Unbundle By Name(w507) -> ("Channel Name"=w505:u16)
          n169 = Index Array(array=w506, index=w505) -> (element=w504:string)
        }
        n170 = call "Head Co-ordinates 2.vi"("3D Type and Co-ordinate System"=T8."Acceleration in Space", "Sample Rate"=w457, "Array"=w477) -> ("Channel List"=w465:string[], "3D Output"=w476:dbl[][])  [unwired: 3 in]
        n171 = Build Array (concatenate)(w467, w466, w465, w464, w463, w462, w459, string[] [" "] ("Input Array")) -> (w461:string[])
        n172 = Build Array (concatenate)(w478, w477, w476, w475, w474, w473, w458) -> (w472:dbl[][])
        n173 = Bundle By Name(cluster=w481, "All Data.Data Channels"=w472, "Data File.Sample Rate"=w457, "All Data.Channel List"=w461) -> (w471:T9)
        n174 = Unbundle By Name(w471) -> ("All Data"=w454:T1)
        n175 = local write "All Data"(w454) -> ()
      }
      frame "Export Channels" {
        n176 = Unbundle By Name(w535) -> ("Data File.Sample Rate"=w536:i32, "All Data.Data Channels"=w534:dbl[][], "All Data.Channel List"=w531:string[])
        n177 = property on="Ring" class="Ring (strict)"("Strings []"=w531) -> ()  [unwired: 2 in, 2 out]
        n178 = for {
          tunnel: w534 -> [w546]
          tunnel: "Export Channel List" -> [w543] mode=indexing
          tunnel: [w545] -> w532 mode=indexing
          tunnel: w531 -> [w544]
          tunnel: [w542] -> w530 mode=indexing
          n179 = Index Array(array=w544, index=w543) -> (element=w542:string)
          n180 = Index Array(array=w546, index (row)=w543) -> (element=w545:dbl[])  [unwired: 1 in]
        }
        n181 = local read "Data Export"() -> (w538:T1)
        n182 = Bundle By Name(cluster=w538, "Sample Rate"=w536, "Data Channels"=w532, "Channel List"=w530) -> (→"Data Export":T1)
      }
      frame "Stop" {
      }
      frame "Quit", Default {
      }
    }
  }
